vi "Read GALVO Calibration File (SubVI).vi"() -> (3 "GALVO Cal Data":T1)   [LabVIEW 2020]
uses:
  Controls (HOST)/IR GALVO Cal Data.ctl
  <vilib>/Utility/file.llb/Read Delimited Spreadsheet (DBL).vi
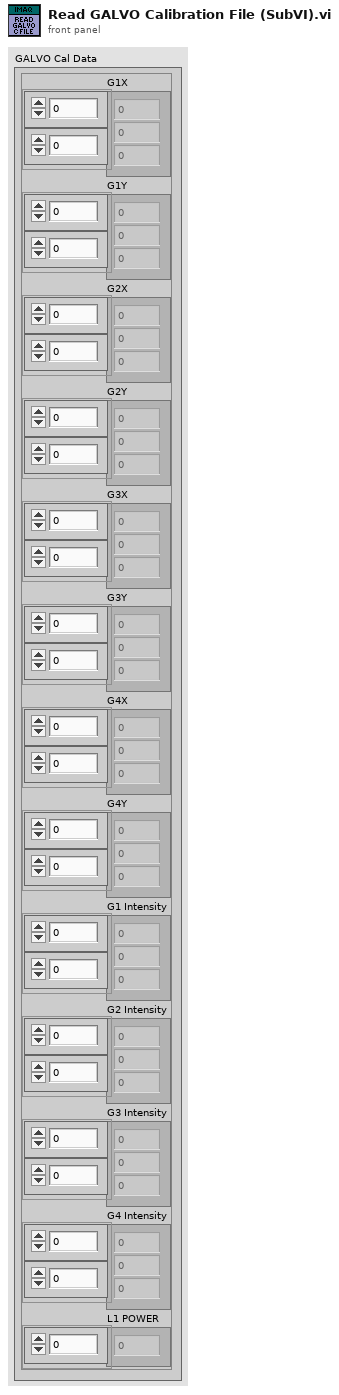
[diagram p1: front panel]
types:
  T1 = typedef "IR GALVO Cal Data.ctl" = cluster{"G1X":dbl[][], "G1Y":dbl[][], "G2X":dbl[][], "G2Y":dbl[][], "G3X":dbl[][], "G3Y":dbl[][], "G4X":dbl[][], "G4Y":dbl[][], "G1 Intensity":dbl[][], "G2 Intensity":dbl[][], "G3 Intensity":dbl[][], "G4 Intensity":dbl[][], "L1 POWER":dbl[]}
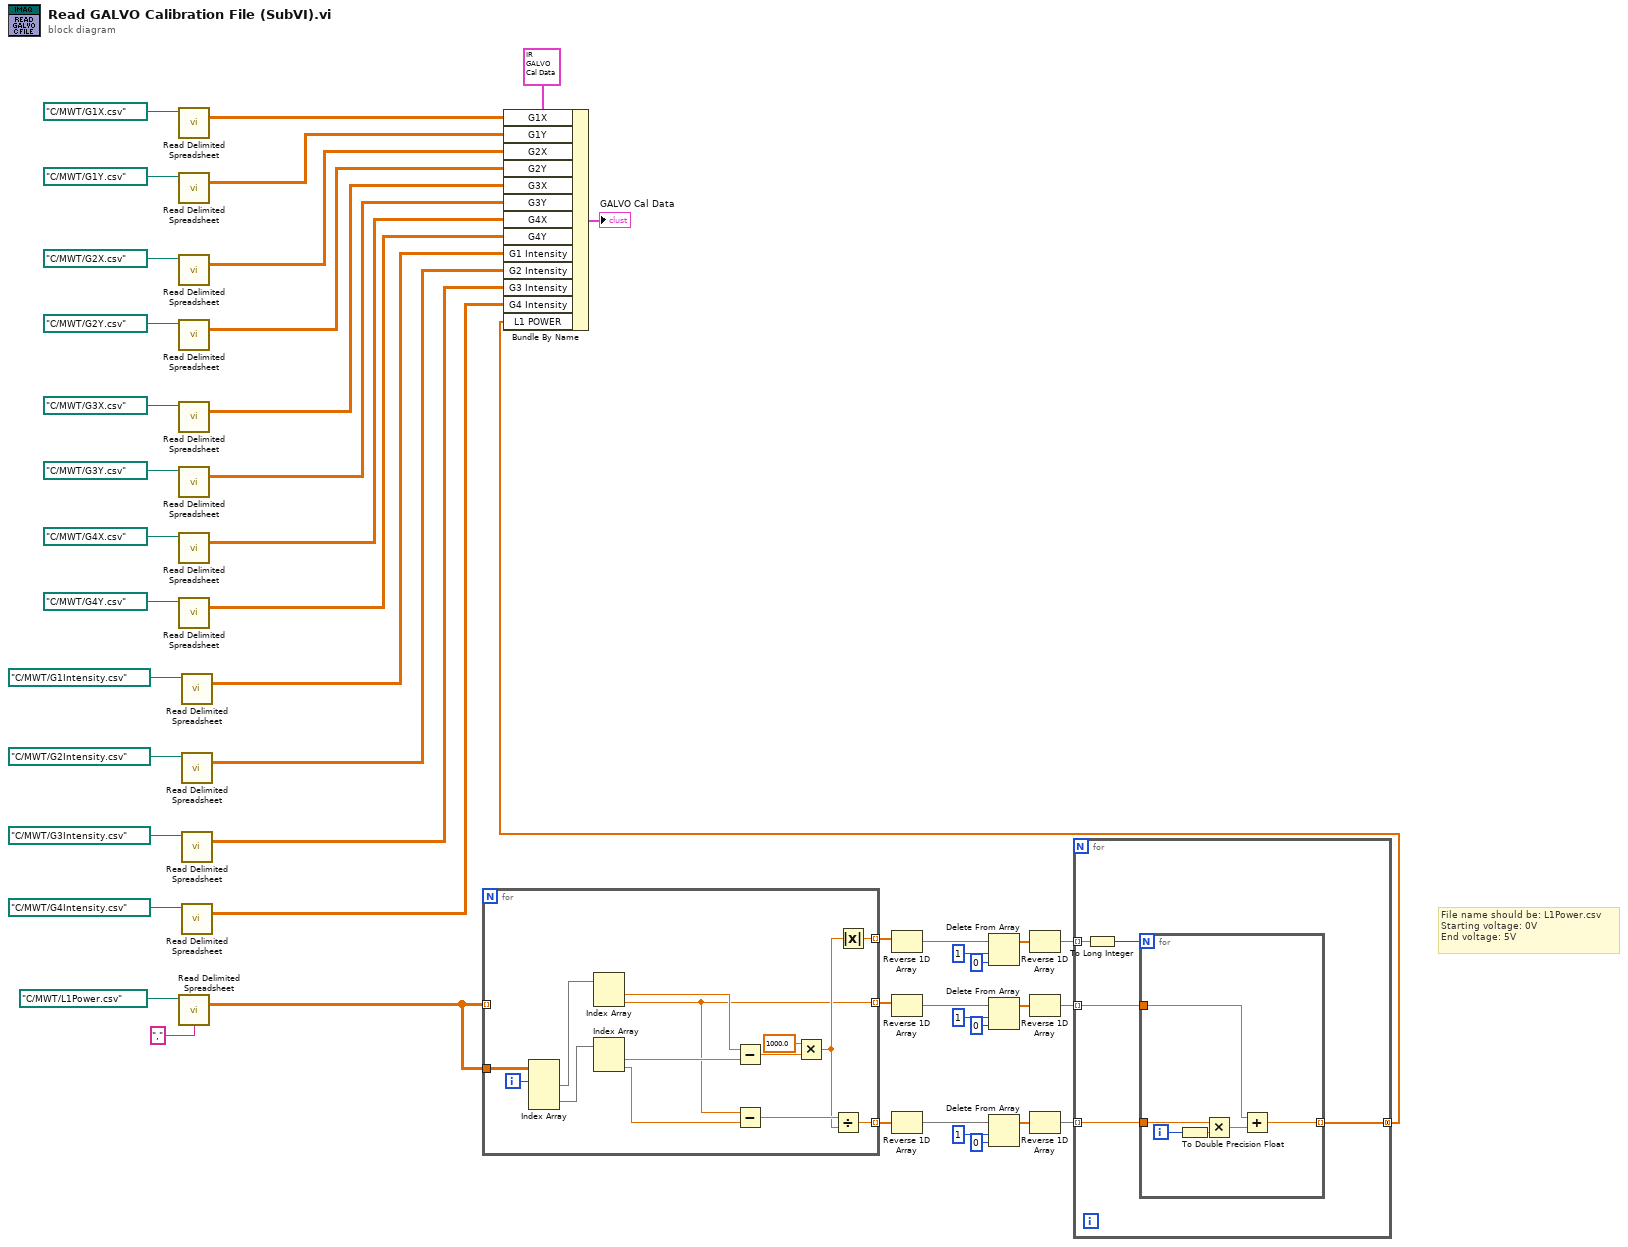
[diagram p0: block diagram]
diagram:
  # "File name should be: L1Power.csv\nStarting voltage: 0V\nEnd voltage: 5V"
  n1 = call-poly <vilib>:"Read Delimited Spreadsheet.vi"("file path (dialog if empty)"=path "C:/MWT/G1X.csv") -> ("all rows"=w47:dbl[][])  [unwired: 9 in, 5 out]
  n2 = call-poly <vilib>:"Read Delimited Spreadsheet.vi"("file path (dialog if empty)"=path "C:/MWT/G1Y.csv") -> ("all rows"=w48:dbl[][])  [unwired: 9 in, 5 out]
  n3 = call-poly <vilib>:"Read Delimited Spreadsheet.vi"("file path (dialog if empty)"=path "C:/MWT/G2X.csv") -> ("all rows"=w37:dbl[][])  [unwired: 9 in, 5 out]
  n4 = call-poly <vilib>:"Read Delimited Spreadsheet.vi"("file path (dialog if empty)"=path "C:/MWT/G2Y.csv") -> ("all rows"=w36:dbl[][])  [unwired: 9 in, 5 out]
  n5 = call-poly <vilib>:"Read Delimited Spreadsheet.vi"("file path (dialog if empty)"=path "C:/MWT/G3X.csv") -> ("all rows"=w35:dbl[][])  [unwired: 9 in, 5 out]
  n6 = call-poly <vilib>:"Read Delimited Spreadsheet.vi"("file path (dialog if empty)"=path "C:/MWT/G3Y.csv") -> ("all rows"=w34:dbl[][])  [unwired: 9 in, 5 out]
  n7 = call-poly <vilib>:"Read Delimited Spreadsheet.vi"("file path (dialog if empty)"=path "C:/MWT/G4X.csv") -> ("all rows"=w33:dbl[][])  [unwired: 9 in, 5 out]
  n8 = call-poly <vilib>:"Read Delimited Spreadsheet.vi"("file path (dialog if empty)"=path "C:/MWT/G4Y.csv") -> ("all rows"=w32:dbl[][])  [unwired: 9 in, 5 out]
  n9 = call-poly <vilib>:"Read Delimited Spreadsheet.vi"("file path (dialog if empty)"=path "C:/MWT/L1Power.csv", "delimiter (\\t)"="," ("delimiter (\\t)")) -> ("all rows"=w20:dbl[][])  [unwired: 8 in, 5 out]
  n10 = call-poly <vilib>:"Read Delimited Spreadsheet.vi"("file path (dialog if empty)"=path "C:/MWT/G1Intensity.csv") -> ("all rows"=w26:dbl[][])  [unwired: 9 in, 5 out]
  n11 = call-poly <vilib>:"Read Delimited Spreadsheet.vi"("file path (dialog if empty)"=path "C:/MWT/G2Intensity.csv") -> ("all rows"=w25:dbl[][])  [unwired: 9 in, 5 out]
  n12 = call-poly <vilib>:"Read Delimited Spreadsheet.vi"("file path (dialog if empty)"=path "C:/MWT/G3Intensity.csv") -> ("all rows"=w24:dbl[][])  [unwired: 9 in, 5 out]
  n13 = call-poly <vilib>:"Read Delimited Spreadsheet.vi"("file path (dialog if empty)"=path "C:/MWT/G4Intensity.csv") -> ("all rows"=w23:dbl[][])  [unwired: 9 in, 5 out]
  n14 = for {
    tunnel: w20 -> [_] mode=indexing
    tunnel: w20 -> [w62]
    tunnel: [w57] -> w19 mode=indexing
    tunnel: [w49] -> w12 mode=indexing
    tunnel: [w50] -> w9 mode=indexing
    i -> [w56]
    n15 = Index Array(array=w62, index (row) #1=w56) -> (element #1=w61:dbl[], element #2=w60:dbl[])  [unwired: 3 in]
    n16 = Index Array(array=w61) -> (element #1=w55:dbl, element #2=w49:dbl)  [unwired: 2 in]
    n17 = Index Array(array=w60) -> (element #1=w51:dbl, element #2=w59:dbl)  [unwired: 2 in]
    n18 = Subtract(x=w55, y=w51) -> (x-y=w54:dbl)
    n19 = Subtract(x=w49, y=w59) -> (x-y=w58:dbl)
    n20 = Multiply(x=1000.0, y=w54) -> (x*y=w53:dbl)
    n21 = Divide(x=w58, y=w53) -> (x/y=w57:dbl)
    n22 = Absolute Value(x=w53) -> (abs(x)=w50:dbl)
  }
  n23 = Reverse 1D Array(array=w9) -> (reversed array=w8:dbl[])
  n24 = Reverse 1D Array(array=w12) -> (reversed array=w13:dbl[])
  n25 = Reverse 1D Array(array=w19) -> (reversed array=w18:dbl[])
  n26 = Delete From Array(array=w8, length=1, index=0) -> (array with subset deleted=w6:dbl[])  [unwired: 1 out]
  n27 = Delete From Array(array=w13, length=1, index=0) -> (array with subset deleted=w15:dbl[])  [unwired: 1 out]
  n28 = Delete From Array(array=w18, length=1, index=0) -> (array with subset deleted=w16:dbl[])  [unwired: 1 out]
  n29 = Reverse 1D Array(array=w6) -> (reversed array=w10:dbl[])
  n30 = Reverse 1D Array(array=w15) -> (reversed array=w11:dbl[])
  n31 = Reverse 1D Array(array=w16) -> (reversed array=w5:dbl[])
  n32 = for {
    tunnel: w10 -> [w65] mode=indexing
    tunnel: w11 -> [w66] mode=indexing
    tunnel: w5 -> [w67] mode=indexing
    tunnel: [w63] -> w4 mode=concatenating
    n33 = To Long Integer(number=w65) -> (32bit integer=w64:i32)
    n34 = for {
      N: w64 -> [_]
      tunnel: w67 -> [w73]
      tunnel: w66 -> [w69]
      tunnel: [w68] -> w63 mode=indexing
      i -> [w72]
      n35 = To Double Precision Float(number=w72) -> (double precision float=w71:dbl)
      n36 = Multiply(x=w73, y=w71) -> (x*y=w70:dbl)
      n37 = Add(x=w69, y=w70) -> (x+y=w68:dbl)
    }
  }
  n38 = Bundle By Name(cluster=T1 {"G1X"=[], "G1Y"=[], "G2X"=[], "G2Y"=[], "G3X"=[], "G3Y"=[], "G4X"=[], "G4Y"=[], "G1 Intensity"=[], "G2 Intensity"=[], "G3 Intensity"=[], "G4 Intensity"=[], "L1 POWER"=[]}, "G1X"=w47, "G1Y"=w48, "G2X"=w37, "G2Y"=w36, "G3X"=w35, "G3Y"=w34, "G4X"=w33, "G4Y"=w32, "G1 Intensity"=w26, "G2 Intensity"=w25, "G3 Intensity"=w24, "G4 Intensity"=w23, "L1 POWER"=w4) -> (→"GALVO Cal Data":T1)
